vi "CRYGet Channel Name From ID and Channel.vi"(6 "Audio Driver":u32, 8 "Channel Name":string, 9 "I/O_channel Info":T1[](array[typedef]) {"Coupling" items=["Default"=-1, "RSE"=10083, "NRSE"=10078, "Differential"=10106, "Pseudodifferential"=12529]; "term config" items=["Default"=-1, "RSE"=10083, "NRSE"=10078, "Differential"=10106, "Pseudodifferential"=12529]; "Anti-aliasing Factor (%fs)" format="%.2f"}, 10 "Channel(LR)":u16, 11 "DeviceID":u32) -> (3 "Channel Info":T1={"ID"=0, "Name"="", "Digital"=FALSE, "Input"=FALSE, "Device Name"="", "Hardware Ch ID"=0, "Vmax (V)"=0.0, "Latency (samples)"=0.0, "Sampling Rate (Hz)"=0, "Bit Depth"=0, "Anti-aliasing Factor (%fs)"=0.475, "DAQmx Channel"="", "term config"=-1, "Coupling"=-1, "IEPE en"=FALSE, "ASIOChannel Name"="", "Audio Driver"=0, "ASIOChannel Index"=0} {"Coupling" items=["Default"=-1, "RSE"=10083, "NRSE"=10078, "Differential"=10106, "Pseudodifferential"=12529]; "term config" items=["Default"=-1, "RSE"=10083, "NRSE"=10078, "Differential"=10106, "Pseudodifferential"=12529]; "Anti-aliasing Factor (%fs)" format="%.2f"})   [LabVIEW 2013]
uses:
  Typedef Control/CRYHardware Channel Info.ctl
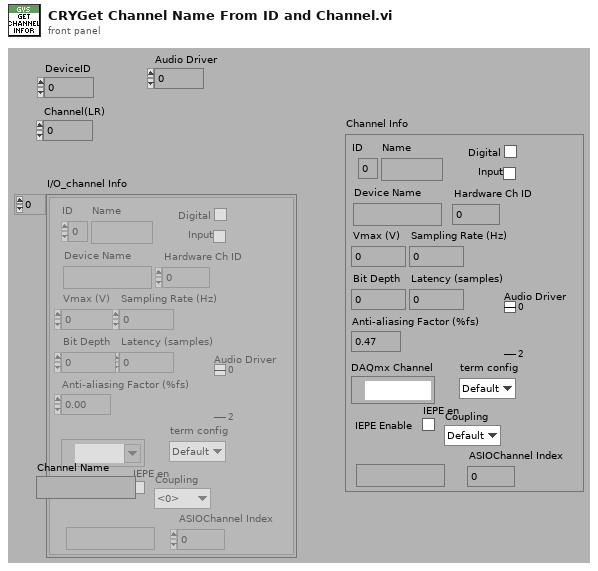
[diagram p1: front panel]
types:
  T1 = typedef "CRYHardware Channel Info.ctl" = cluster{"ID":i32, "Name":string, "Digital":bool, "Input":bool, "Device Name":string, "Hardware Ch ID":u8, "Vmax (V)":dbl, "Latency (samples)":dbl, "Sampling Rate (Hz)":u32, "Bit Depth":u32, "Anti-aliasing Factor (%fs)":sgl, "DAQmx Channel":tag, "term config":i32, "Coupling":i32, "IEPE en":bool, "ASIOChannel Name":string, "Audio Driver":u16, "ASIOChannel Index":u8}
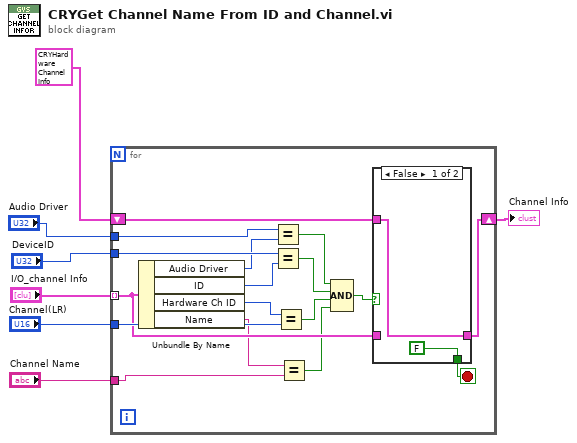
[diagram p0: block diagram]
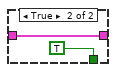
[diagram p2: hidden frame]
diagram:
  n1 = for {
    tunnel: "I/O_channel Info" -> [w15] mode=indexing
    tunnel: "DeviceID" -> [w24]
    tunnel: "Channel(LR)" -> [w21]
    shift-right: [w14] -> w3
    shift-left: T1 {"ID"=0, "Name"="", "Digital"=FALSE, "Input"=FALSE, "Device Name"="", "Hardware Ch ID"=0, "Vmax (V)"=0.0, "Latency (samples)"=0.0, "Sampling Rate (Hz)"=0, "Bit Depth"=0, "Anti-aliasing Factor (%fs)"=0.475, "DAQmx Channel"="", "term config"=0, "Coupling"=-1, "IEPE en"=FALSE, "ASIOChannel Name"="", "Audio Driver"=0, "ASIOChannel Index"=0} ("Channel Info") -> [w16]
    tunnel: "Channel Name" -> [w13]
    tunnel: "Audio Driver" -> [w9]
    stop <- w17 stop-if-true
    n2 = Unbundle By Name(w15) -> ("Audio Driver"=w10:u16, "ID"=w23:i32, "Hardware Ch ID"=w22:u8, "Name"=w12:string)
    n3 = Equal?(x=w9, y=w10) -> (x = y?=w8:bool)
    n4 = Equal?(x=w24, y=w23) -> (x = y?=w20:bool)
    n5 = Equal?(x=w22, y=w21) -> (x = y?=w19:bool)
    n6 = Equal?(x=w12, y=w13) -> (x = y?=w11:bool)
    n7 = Compound Arithmetic op=AND(w8, w20, w19, w11) -> (w18:bool)
    n8 = case shown="False" w18 {
      tunnel: [FALSE TRUE] -> w17
      tunnel: [w25 w27] -> w14
      tunnel: w16 -> [w25 _]
      tunnel: w15 -> [_ w27]
      frame False {
      }
      frame True {
      }
    }
  }
  "Channel Info" <- w3
